vi "isRunning.vi"(8 "error in (no error)":errorcluster, 11 "TaskController in":refnum<class "TaskController.lvclass">) -> (0 "error out":errorcluster, 2 "isRunning":bool, 3 "TaskController out":refnum<class "TaskController.lvclass">)   [LabVIEW 2023, in "TLC_Daemon.lvlib" / "TaskController.lvclass"]
doc: "is the task running?\n_____________________________________\nTLC Daemon 1.0.0.2\nCopyright (c) 2026 Andrea Cadei"
uses:
  TaskController.lvclass
  TaskController.lvclass/TaskController.ctl
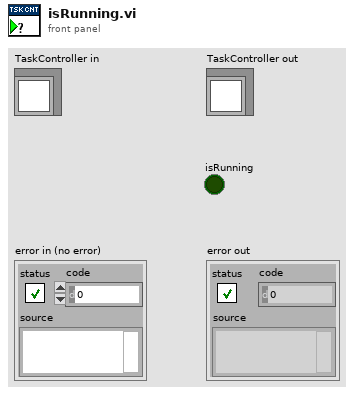
[diagram p1: front panel]
types:
  T1 = typedef "TLC_Daemon.lvlib/TaskController.lvclass/status.ctl" = enum16{"NotReady", "Ready", "Running", "Stopped", "Unknown"}
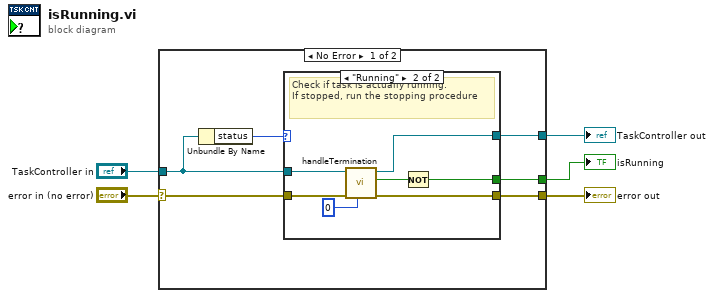
[diagram p0: block diagram]
diagram:
  n1 = case shown="No Error" "error in (no error)" {
    selector: "error in (no error)" -> [w10 w22]
    tunnel: [w11 w22] -> w4
    tunnel: [w8 w21] -> w2
    tunnel: "TaskController in" -> [w7 w21]
    tunnel: [w9 _] -> w1
    frame No Error {
      n2 = Unbundle By Name(w7) -> ("status"=w6:T1)
      n3 = case shown="\"Running\"" w6 {
        tunnel: [w12 w20] -> w11
        tunnel: w10 -> [w12 w19]
        tunnel: [_ w18] -> w9
        tunnel: [w13 w17] -> w8
        tunnel: w7 -> [w13 w16]
        frame Default {
        }
        frame "Running" {
          # "Check if task is actually running.\nIf stopped, run the stopping procedure"
          n4 = call "handleTermination.vi"("timeout[ms]"=0, "error in (no error)"=w19, "TaskController in"=w16) -> ("error out"=w20:errorcluster, "terminated?"=w14:bool, "TaskController out"=w17:refnum<class "TaskController.lvclass">)  [unwired: 6 in]
          n5 = Not(x=w14) -> (.not. x?=w18:bool)
        }
      }
    }
    frame Error {
    }
  }
  "error out" <- w4
  "TaskController out" <- w2
  "isRunning" <- w1
